vi "PrepareAndSendStartAcq.vi"(0 "CameraController in":refnum<class "CameraController.lvclass">, 1 "SingleStack?":bool, 2 "StreamToDisk?":bool, 3 "Alert when finish?":bool, 4 "Mode":T1 items=["Idle", "Snap", "Live", "Capturing", ""], 5 "error in (no error)":errorcluster, 6 "Save Path":path, 7 "File Suffix":string) -> (14 "CameraController out":refnum<class "CameraController.lvclass">, 19 "error out":errorcluster)   [LabVIEW 2020, in "CameraController.lvlib" / "CameraController.lvclass"]
uses:
  CameraController.lvclass
  C:/Program Files/National Instruments/LabVIEW 2020/vi.lib/ActorFramework/Actor/Actor.lvclass
  Model/Hardware Layer/Real Hardware/Camera_Prime95B/Camera_Prime95B/Controls/Camera Status.ctl
  Model/Hardware Layer/Real Hardware/Camera_Prime95B/Camera_Prime95B/Controls/AcquisitionParams.ctl
  Model/Hardware Abstraction Layer/Component/Device/Device/DataExchange.ctl
  <vilib>/ActorFramework/Actor/Actor.lvclass/Actor.ctl
  Model/Hardware Abstraction Layer/Component/Device/Device Messages/StartSequenceAcquisition Msg/StartSequenceAcquisition Msg.lvclass/StartSequenceAcquisition Msg.ctl
  <vilib>/ActorFramework/Message Enqueuer/Message Enqueuer.lvclass/Message Enqueuer.ctl
  <vilib>/ActorFramework/Message Enqueuer/Enqueue.vi
  Model/Hardware Abstraction Layer/Component/Device/Device Messages/StartSequenceAcquisition Msg/StartSequenceAcquisition Msg.lvclass
  C:/Program Files/National Instruments/LabVIEW 2020/vi.lib/ActorFramework/Message/Message.lvclass
  <vilib>/ActorFramework/Message Priority Queue/Priority Enqueue.vi
  <vilib>/ActorFramework/Actor/Actor.lvclass
  Model/Hardware Layer/Real Hardware/Camera_Prime95B/Camera_Prime95B/Camera_Prime95B.lvclass
  Interface/DataListener/DataListener.lvclass
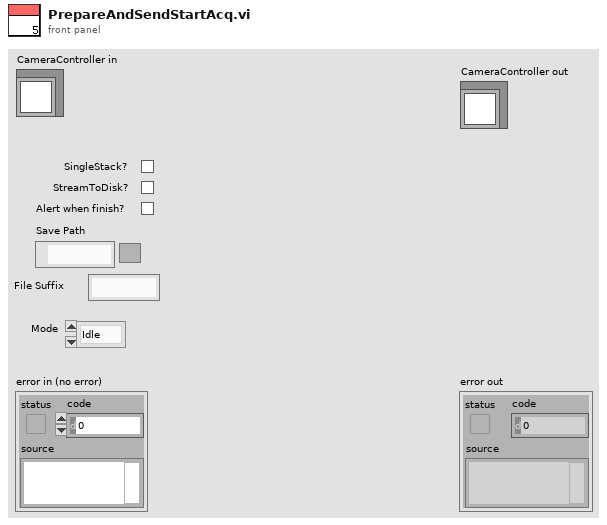
[diagram p1: front panel]
types:
  T1 = typedef "Camera_Prime95B.lvlib/Camera_Prime95B.lvclass/Camera Status.ctl" = i32
  T2 = typedef "DataListener.lvclass/DataExchange.ctl" = cluster{"Source":string, "Destination":string, "Description":string, "value":variant}
  T3 = typedef "Camera_Prime95B.lvlib/Camera_Prime95B.lvclass/AcquisitionParams.ctl" = cluster{"Acq Mode":T1, "Save Path":path, "Stream Save Path":path, "SingleStack?":bool, "StreamToDisk?":bool, "Alert when finish?":bool}
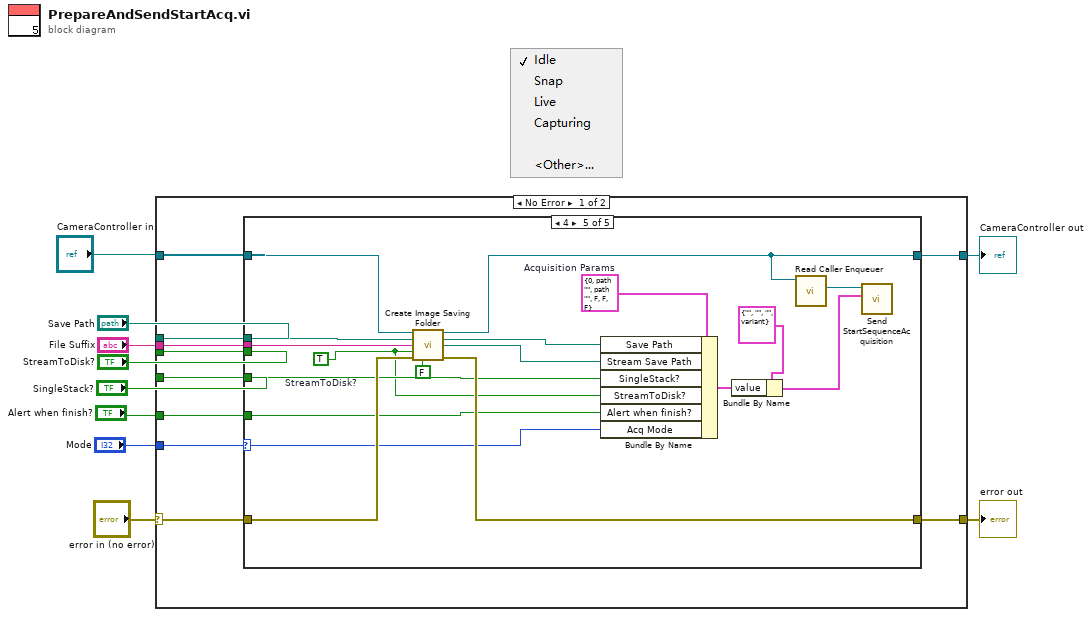
[diagram p0: block diagram]
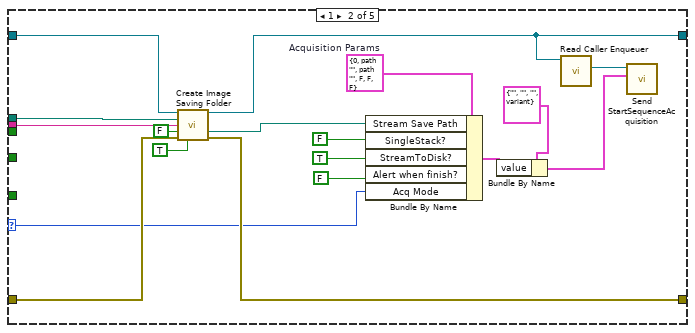
[diagram p3: hidden frame]
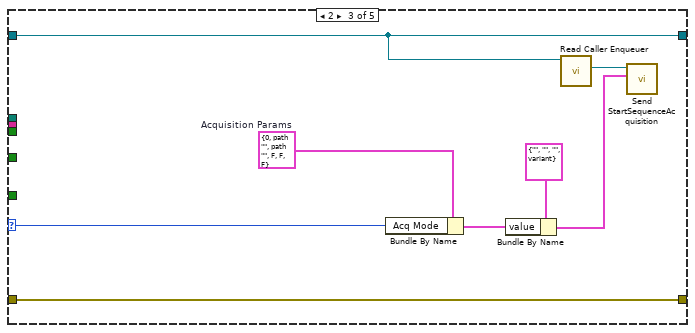
[diagram p4: hidden frame]
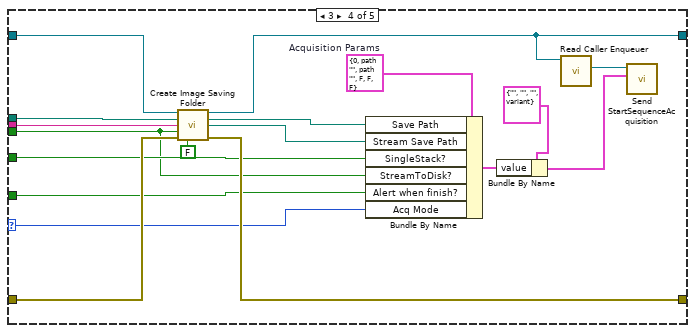
[diagram p5: hidden frame]
diagram:
  n1 = case shown="No Error" "error in (no error)" {
    selector: "error in (no error)" -> [w18 w86]
    tunnel: [w17 w86] -> w9
    tunnel: [w19 w85] -> w7
    tunnel: "CameraController in" -> [w20 w85]
    tunnel: "StreamToDisk?" -> [w13 _]
    tunnel: "Save Path" -> [w16 _]
    tunnel: "File Suffix" -> [w15 _]
    tunnel: "SingleStack?" -> [w14 _]
    tunnel: "Alert when finish?" -> [w12 _]
    tunnel: "Mode" -> [w11 _]
    frame No Error {
      n2 = case shown="4" w11 {
        selector: w11 -> [_ w29 w41 w50 w69]
        tunnel: w20 -> [w22 w39 w47 w65 w83]
        tunnel: [w22 w38 w47 w64 w82] -> w19
        tunnel: w18 -> [w21 w37 w46 w63 w81]
        tunnel: [w21 w36 w46 w62 w80] -> w17
        tunnel: w16 -> [_ w35 _ w61 w79]
        tunnel: w15 -> [_ w34 _ w60 w78]
        tunnel: w14 -> [_ _ _ w56 w74]
        tunnel: w13 -> [_ _ _ w55 _]
        tunnel: w12 -> [_ _ _ w54 w73]
        frame 0, Default {
        }
        frame 1 {
          w33 = T3 {"Acq Mode"=0, "Save Path"=path "", "Stream Save Path"=path "", "SingleStack?"=FALSE, "StreamToDisk?"=FALSE, "Alert when finish?"=FALSE}  # Acquisition Params
          n3 = call-dynamic "Create Image Saving Folder.vi"("Camera Prime95B Controller in"=w39, "Save Path"=w35, "File suffix"=w34, "StreamToDisk?"=FALSE, "error in (no error)"=w37, "SnapShot?"=TRUE) -> ("Camera Prime95B Controller out"=w38:refnum<class "CameraController.lvclass">, "Snap Shot Path"=w24:path, "error out"=w36:errorcluster)  [unwired: 5 in, 2 out]
          n4 = Bundle By Name(cluster=w33, "Stream Save Path"=w24, "SingleStack?"=FALSE, "StreamToDisk?"=TRUE, "Alert when finish?"=FALSE, "Acq Mode"=w29) -> (w32:T3)
          n5 = Bundle By Name(cluster=T2 {"Source"="", "Destination"="", "Description"="", "value"=variant} ("input cluster"), "value"=w32) -> (w30:T2)
          n6 = call <vilib>:"Read Caller Enqueuer.vi"("Actor"=w38) -> ("Caller Enqueuer"=w40:refnum<class "Message Enqueuer.lvclass">)  [unwired: 10 in]
          n7 = call "Send StartSequenceAcquisition.vi"("DataExchange"=w30, "Message Enqueuer"=w40) -> ()  [unwired: 8 in, 2 out]
        }
        frame 2 {
          w45 = T3 {"Acq Mode"=0, "Save Path"=path "", "Stream Save Path"=path "", "SingleStack?"=FALSE, "StreamToDisk?"=FALSE, "Alert when finish?"=FALSE}  # Acquisition Params
          n8 = Bundle By Name(cluster=w45, "Acq Mode"=w41) -> (w44:T3)
          n9 = Bundle By Name(cluster=T2 {"Source"="", "Destination"="", "Description"="", "value"=variant} ("input cluster"), "value"=w44) -> (w42:T2)
          n10 = call <vilib>:"Read Caller Enqueuer.vi"("Actor"=w47) -> ("Caller Enqueuer"=w48:refnum<class "Message Enqueuer.lvclass">)  [unwired: 10 in]
          n11 = call "Send StartSequenceAcquisition.vi"("DataExchange"=w42, "Message Enqueuer"=w48) -> ()  [unwired: 8 in, 2 out]
        }
        frame 3 {
          w58 = T3 {"Acq Mode"=0, "Save Path"=path "", "Stream Save Path"=path "", "SingleStack?"=FALSE, "StreamToDisk?"=FALSE, "Alert when finish?"=FALSE}  # Acquisition Params
          n12 = call-dynamic "Create Image Saving Folder.vi"("Camera Prime95B Controller in"=w65, "Save Path"=w61, "File suffix"=w60, "StreamToDisk?"=w55, "error in (no error)"=w63, "SnapShot?"=FALSE) -> ("Camera Prime95B Controller out"=w64:refnum<class "CameraController.lvclass">, "Saving Path"=w59:path, "Stream Saving Path"=w57:path, "error out"=w62:errorcluster)  [unwired: 5 in, 1 out]
          n13 = Bundle By Name(cluster=w58, "Save Path"=w59, "Stream Save Path"=w57, "SingleStack?"=w56, "StreamToDisk?"=w55, "Alert when finish?"=w54, "Acq Mode"=w50) -> (w53:T3)
          n14 = Bundle By Name(cluster=T2 {"Source"="", "Destination"="", "Description"="", "value"=variant} ("input cluster"), "value"=w53) -> (w51:T2)
          n15 = call <vilib>:"Read Caller Enqueuer.vi"("Actor"=w64) -> ("Caller Enqueuer"=w66:refnum<class "Message Enqueuer.lvclass">)  [unwired: 10 in]
          n16 = call "Send StartSequenceAcquisition.vi"("DataExchange"=w51, "Message Enqueuer"=w66) -> ()  [unwired: 8 in, 2 out]
        }
        frame 4 {
          w67 = TRUE  # StreamToDisk?
          w76 = T3 {"Acq Mode"=0, "Save Path"=path "", "Stream Save Path"=path "", "SingleStack?"=FALSE, "StreamToDisk?"=FALSE, "Alert when finish?"=FALSE}  # Acquisition Params
          n17 = call-dynamic "Create Image Saving Folder.vi"("Camera Prime95B Controller in"=w83, "Save Path"=w79, "File suffix"=w78, "StreamToDisk?"=w67, "error in (no error)"=w81, "SnapShot?"=FALSE) -> ("Camera Prime95B Controller out"=w82:refnum<class "CameraController.lvclass">, "Saving Path"=w77:path, "Stream Saving Path"=w75:path, "error out"=w80:errorcluster)  [unwired: 5 in, 1 out]
          n18 = Bundle By Name(cluster=w76, "Save Path"=w77, "Stream Save Path"=w75, "SingleStack?"=w74, "StreamToDisk?"=w67, "Alert when finish?"=w73, "Acq Mode"=w69) -> (w72:T3)
          n19 = Bundle By Name(cluster=T2 {"Source"="", "Destination"="", "Description"="", "value"=variant} ("input cluster"), "value"=w72) -> (w70:T2)
          n20 = call <vilib>:"Read Caller Enqueuer.vi"("Actor"=w82) -> ("Caller Enqueuer"=w84:refnum<class "Message Enqueuer.lvclass">)  [unwired: 10 in]
          n21 = call "Send StartSequenceAcquisition.vi"("DataExchange"=w70, "Message Enqueuer"=w84) -> ()  [unwired: 8 in, 2 out]
        }
      }
    }
    frame Error {
    }
  }
  "error out" <- w9
  "CameraController out" <- w7
